vi "Gif.GraphicControlExtension.vi"(0 "data":string, 9 "offset":i32, 11 "error in (no error)":errorcluster) -> (4 "data out":string, 6 "GraphicControlExtension":T1, 10 "offset out":i32, 15 "error out":errorcluster)   [LabVIEW 2011]
uses:
  Gif.GraphicControlExtension.ctl
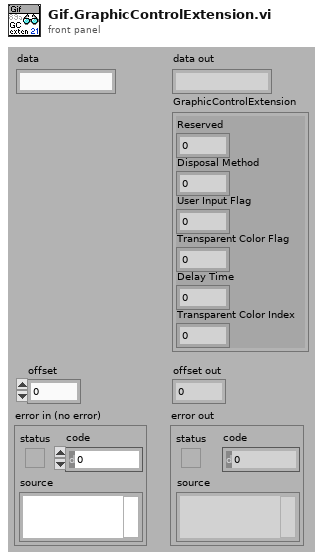
[diagram p1: front panel]
types:
  T1 = typedef "Gif.GraphicControlExtension.ctl" = cluster{"Reserved":u8, "Disposal Method":u8, "User Input Flag":u8, "Transparent Color Flag":u8, "Delay Time":u16, "Transparent Color Index":u8}
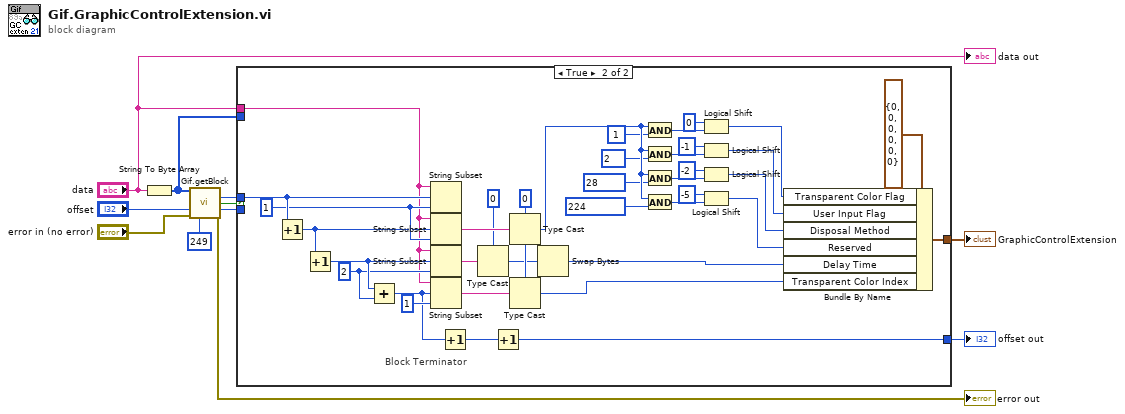
[diagram p0: block diagram]
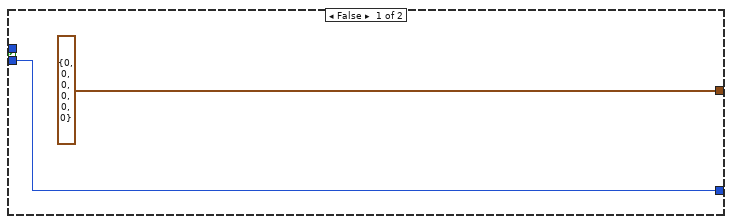
[diagram p2: hidden frame]
diagram:
  n1 = String To Byte Array(string="data") -> (unsigned byte array=w8:u8[])
  n2 = call "Gif.getBlock.vi"("data"=w8, "offset"="offset", "error in (no error)"="error in (no error)", "label"=u8 249 ("element")) -> ("pos offset"=w9:i32, "found?"=w10:bool, "offset out"=w7:i32, "error out"=→"error out":errorcluster)  [unwired: 8 out]
  n3 = case shown="True" w10 {
    tunnel: w9 -> [_ w50]
    tunnel: "data" -> [_ w45]
    tunnel: w8 -> [_ _]
    tunnel: w7 -> [w13 _]
    tunnel: [w13 w35] -> w6
    tunnel: [T1 {"Reserved"=0, "Disposal Method"=0, "User Input Flag"=0, "Transparent Color Flag"=0, "Delay Time"=0, "Transparent Color Index"=0} ("GraphicControlExtension") w28] -> w1
    frame False {
    }
    frame True {
      w40 = u8 0 ("length (rest)")
      w46 = 2 ("length (rest)")
      w49 = 1 ("length (rest)")
      # "Block Terminator"
      n4 = Increment(x=w50) -> (x+1=w48:i32)
      n5 = Increment(x=w48) -> (x+1=w47:i32)
      n6 = Add(x=w47, y=w46) -> (x+y=w37:i32)
      n7 = String Subset(string=w45, offset (0)=w50, length (rest)=w49) -> ()  [unwired: 1 out]
      n8 = String Subset(string=w45, offset (0)=w48, length (rest)=w49) -> (substring=w43:string)
      n9 = String Subset(string=w45, offset (0)=w47, length (rest)=w46) -> (substring=w42:string)
      n10 = String Subset(string=w45, offset (0)=w37, length (rest)=1 ("length (rest)")) -> (substring=w41:string)
      n11 = Increment(x=w37) -> (x+1=w36:i32)
      n12 = Type Cast(type=u16 0 ("length (rest)"), x=w42) -> (*(type *) &x=w27:u16)
      n13 = Increment(x=w36) -> (x+1=w35:i32)
      n14 = Type Cast(type=w40, x=w43) -> (*(type *) &x=w38:u8)
      n15 = Type Cast(type=w40, x=w41) -> (*(type *) &x=w31:u8)
      n16 = Swap Bytes(anything=w27) -> (byte swapped=w26:u16)
      n17 = And(x=w38, y=u8 1 ("length (rest)")) -> (x .and. y?=w20:u8)
      n18 = And(x=w38, y=u8 2 ("length (rest)")) -> (x .and. y?=w19:u8)
      n19 = And(x=w38, y=u8 28 ("length (rest)")) -> (x .and. y?=w18:u8)
      n20 = And(x=w38, y=u8 224 ("length (rest)")) -> (x .and. y?=w21:u8)
      n21 = Logical Shift(y=0, x=w20) -> (x << y=w33:u8)
      n22 = Logical Shift(y=-1, x=w19) -> (x << y=w32:u8)
      n23 = Logical Shift(y=-2, x=w18) -> (x << y=w30:u8)
      n24 = Logical Shift(y=-5, x=w21) -> (x << y=w29:u8)
      n25 = Bundle By Name(cluster=T1 {"Reserved"=0, "Disposal Method"=0, "User Input Flag"=0, "Transparent Color Flag"=0, "Delay Time"=0, "Transparent Color Index"=0} ("GraphicControlExtension"), "Transparent Color Flag"=w33, "User Input Flag"=w32, "Disposal Method"=w30, "Reserved"=w29, "Delay Time"=w26, "Transparent Color Index"=w31) -> (w28:T1)
    }
  }
  "offset out" <- w6
  "GraphicControlExtension" <- w1
  "data out" <- "data"
